vi "Vision Test10.vi"() -> ()   [LabVIEW 2016]
uses:
  <vilib>/userdefined/High Color/IMAQdx.ctl
  <vilib>/vision/driver/IMAQdx.llb/IMAQdx Camera Control Mode.ctl
  <vilib>/vision/driver/NI_Vision_Acquisition_Software.lvlib
panel:
  out "Like":i32
  out "Like":bool
  out "Image 2":T1(plugin-control)
  in  "Session In":T2
  out "C":i32
  out "C":bool
  out "Palm":i32
  out "Palm":bool
  out "Number of Matches (Two Fingers)  2":i32
  out "2 Fingers 2":bool
  out "Number of Matches (Two Fingers)":i32
  out "2 Fingers":bool
  out "Number of Matches (Five Fingers)":i32
  out "5 Fingers":bool
  out "Image":T1(plugin-control)
  out "Frame Rate":dbl
  in  "Stop (F)":bool
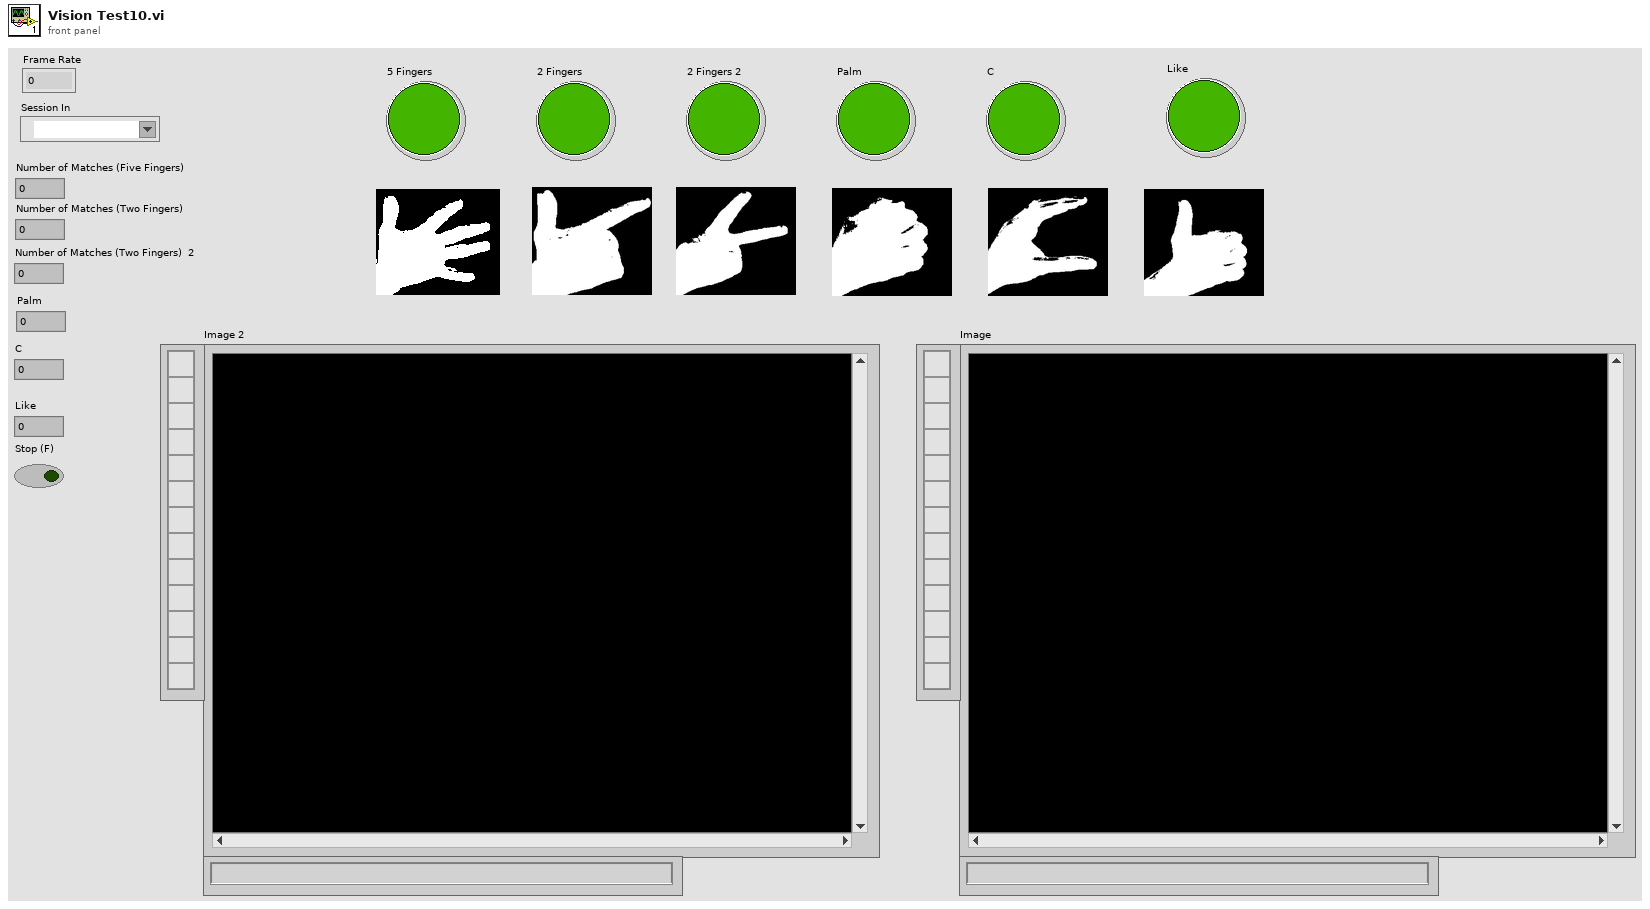
[diagram p1: front panel]
types:
  T1 = typedef "IMAQ Image.ctl" = refnum<image>
  T2 = typedef "IMAQdx.ctl" = refnum<k21>
  T3 = typedef "NI_Vision_Acquisition_Software.lvlib/IMAQdx Camera Control Mode.ctl" = enum32{"Controller", "Listener"}
  T4 = typedef "Image Type" = u32
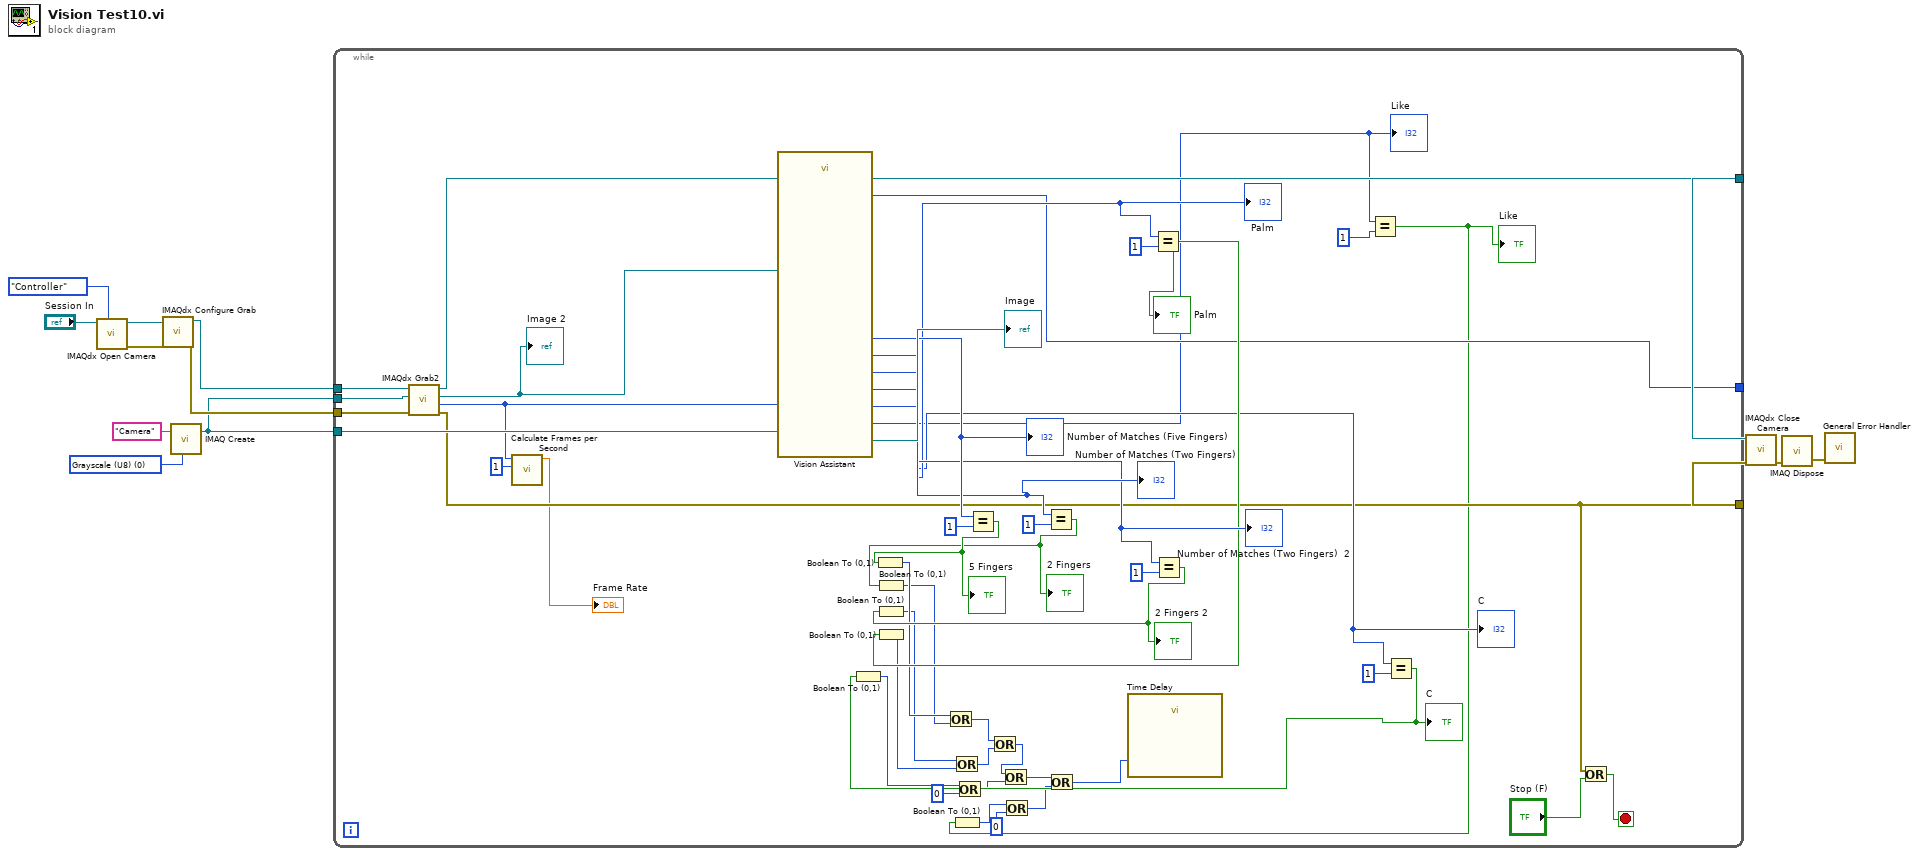
[diagram p0: block diagram]
diagram:
  w12 = T4 0 items=["Grayscale (U8)", "Grayscale (I16)", "Grayscale (SGL)", "Complex (CSG)", "RGB (U32)", "HSL (U32)", "RGB (U64)", "Grayscale (U16)"] ("Image Type")
  n1 = call <vilib>:"IMAQdx Open Camera.vi"("Camera Control Mode"=IMAQdx_Camera_Control_Mode."Controller", "Session In"="Session In") -> ("error out"=w6:errorcluster, "Session Out"=w7:T2)  [unwired: 8 in]
  n2 = call <vilib>:"IMAQdx Configure Grab.vi"("error in"=w6, "Session In"=w7) -> ("error out"=w4:errorcluster, "Session Out"=w5:T2)  [unwired: 8 in]
  n3 = call "IMAQ Create"("Image Name"="Camera", "Image Type"=w12) -> ("New Image"=w3:T1)  [unwired: 3 in, 1 out]
  n4 = while {
    tunnel: w3 -> [w59]
    tunnel: w5 -> [w32]
    tunnel: w4 -> [w31]
    tunnel: w3 -> [w30]
    tunnel: [w27] -> w2
    tunnel: [w26] -> w1
    tunnel: [w24] -> _
    stop <- w28 stop-if-true
    n5 = call <vilib>:"IMAQdx Grab2.vi"("error in"=w31, "Image In"=w30, "Session In"=w32) -> ("error out"=w26:errorcluster, "Buffer Number Out"=w24:u32, "Image Out"=w22:T1, "Session Out"=w27:T2)  [unwired: 5 in]
    "Image 2" <- w22
    n6 = call <vilib>:"Calculate Frames per Second.vi"("Update Interval (ms)"=u32 1, "Buffer Number"=w24) -> ("Acquired Frames/s"=→"Frame Rate":dbl)  [unwired: 7 in, 2 out]
    n7 = call "Vision Assistant"("Image In"=w22, "Image Dst"=w59) -> ("Image Out"=→"Image":T1, "Number of Matches (Pattern Matching 1)"=w56:i32, "Number of Matches (Pattern Matching 2)"=w54:i32, "Number of Matches (Pattern Matching 3)"=w52:i32, "Number of Matches (Pattern Matching 5)"=w38:i32, "Number of Matches (Pattern Matching 4)"=w50:i32, "Number of Matches (Pattern Matching 6)"=w21:i32)  [unwired: 18 in, 1 out]
    "Number of Matches (Five Fingers)" <- w56
    "Number of Matches (Two Fingers)" <- w54
    "Number of Matches (Two Fingers)  2" <- w52
    "Palm" <- w50
    "C" <- w38
    "Like" <- w21
    n8 = Equal?(x=w56, y=1) -> (x = y?=w49:bool)
    "5 Fingers" <- w49
    n9 = Boolean To (0,1)(Boolean=w49) -> (0, 1=w45:i16)
    n10 = Equal?(x=w54, y=1) -> (x = y?=w48:bool)
    "2 Fingers" <- w48
    n11 = Boolean To (0,1)(Boolean=w48) -> (0, 1=w44:i16)
    n12 = Or(x=w45, y=w44) -> (x .or. y?=w41:i16)
    n13 = Equal?(x=w50, y=1) -> (x = y?=w46:bool)
    "Palm" <- w46
    n14 = Boolean To (0,1)(Boolean=w46) -> (0, 1=w42:i16)
    n15 = Equal?(x=w52, y=1) -> (x = y?=w47:bool)
    "2 Fingers 2" <- w47
    n16 = Boolean To (0,1)(Boolean=w47) -> (0, 1=w43:i16)
    n17 = Or(x=w43, y=w42) -> (x .or. y?=w40:i16)
    n18 = Or(x=w41, y=w40) -> (x .or. y?=w33:i16)
    n19 = Equal?(x=w21, y=1) -> (x = y?=w18:bool)
    "Like" <- w18
    n20 = Boolean To (0,1)(Boolean=w18) -> (0, 1=w19:i16)
    n21 = Or(x=w19, y=i16 0) -> (x .or. y?=w16:i16)
    n22 = Equal?(x=w38, y=1) -> (x = y?=w37:bool)
    "C" <- w37
    n23 = Boolean To (0,1)(Boolean=w37) -> (0, 1=w36:i16)
    n24 = Or(x=w36, y=i16 0) -> (x .or. y?=w34:i16)
    n25 = Or(x=w33, y=w34) -> (x .or. y?=w17:i16)
    n26 = Or(x=w17, y=w16) -> (x .or. y?=w14:i16)
    n27 = call "Time Delay"("Delay Time (s)"=w14) -> ()  [unwired: 10 in, 1 out]
    n28 = Or(x=w26, y="Stop (F)") -> (x .or. y?=w28:bool)
  }
  n29 = call <vilib>:"IMAQdx Close Camera.vi"("error in"=w1, "Session In"=w2) -> ("error out"=w11:errorcluster)  [unwired: 9 in]
  n30 = call "IMAQ Dispose"("error in (no error)"=w11) -> ("error out"=w10:errorcluster)  [unwired: 5 in]
  n31 = call <vilib>:"General Error Handler.vi"("error in (no error)"=w10) -> ()  [unwired: 10 in, 5 out]
